vi "Refresh Channel Pairing by Ref.vi"(8 "error in (no error)":errorcluster, 10 "engine":refnum<data-value>, 11 "E2E editor node in":refnum<data-value>) -> (0 "error out":errorcluster, 2 "engine out":refnum<data-value>, 3 "E2E editor node out":refnum<data-value>)   [LabVIEW 2015, in "E2E Tag Exchange editor node.lvclass"]
uses:
  E2E Tag Exchange editor node.lvclass
  <vilib>/NI/DCAF/Tag Editor Core/Configuration Editor/Classes/Engine Parent/Engine Parent Editor Node.lvclass
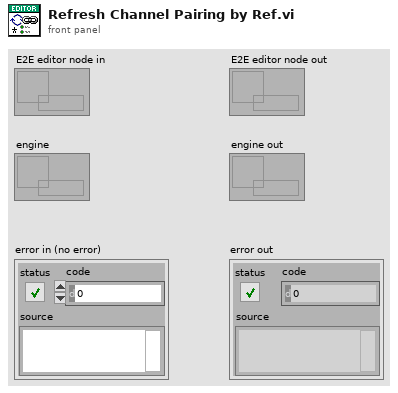
[diagram p1: front panel]
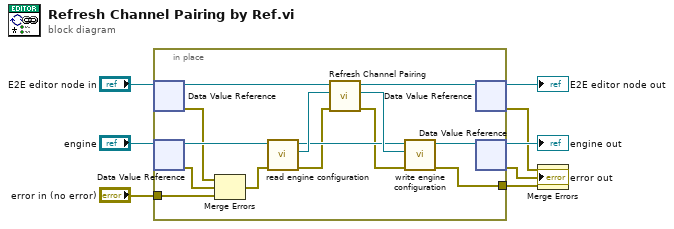
[diagram p0: block diagram]
diagram:
  n1 = in-place {
    in-place-border: "error in (no error)" -> [w14]
    in-place-border: [w10] -> w4
    n2 = in-place-dvr #1("E2E editor node in") -> (w23:refnum<class "E2E Tag Exchange editor node.lvclass">, w12:errorcluster)
    n3 = in-place-dvr #2("engine") -> (w21:refnum<class "Engine Parent Editor Node.lvclass">, w13:errorcluster)
    n4 = Merge Errors(w12, w13, w14) -> (w11:errorcluster)
    n5 = call <vilib>:"read engine configuration.vi"("error in"=w11, "Engine Parent Editor Node in"=w21) -> ("error out"=w16:errorcluster, "engine configuration"=w20:refnum<class "engine configuration.lvclass">, "Engine Parent Editor Node out"=w18:refnum<class "Engine Parent Editor Node.lvclass">)  [unwired: 7 in]
    n6 = call "Refresh Channel Pairing.vi"("error in (no error)"=w16, "engine configuration in"=w20, "E2E editor node in"=w23) -> ("error out"=w15:errorcluster, "engine configuration out"=w19:refnum<class "engine configuration.lvclass">, "E2E editor node out"=w22:refnum<class "E2E Tag Exchange editor node.lvclass">)  [unwired: 6 in]
    n7 = call <vilib>:"write engine configuration.vi"("error in"=w15, "engine configuration"=w19, "Engine Parent Editor Node in"=w18) -> ("error out"=w10:errorcluster, "Engine Parent Editor Node out"=w17:refnum<class "Engine Parent Editor Node.lvclass">)  [unwired: 7 in]
    n8 = in-place-dvr #1(w22) -> (→"E2E editor node out":refnum<data-value>, w2:errorcluster)
    n9 = in-place-dvr #2(w17) -> (→"engine out":refnum<data-value>, w3:errorcluster)
  }
  n10 = Merge Errors(w2, w3, w4) -> (→"error out":errorcluster)
